vi "EEGteam5.vi"() -> ()   [LabVIEW 2011]
panel:
  in  "stop":bool
  out "After_notch Graph":dynamicdata(graph)
  out "Unfiltered":dynamicdata(graph)
  out "Beta Graph 2":dynamicdata(graph)
  out "Alpha Graph":dynamicdata(graph)
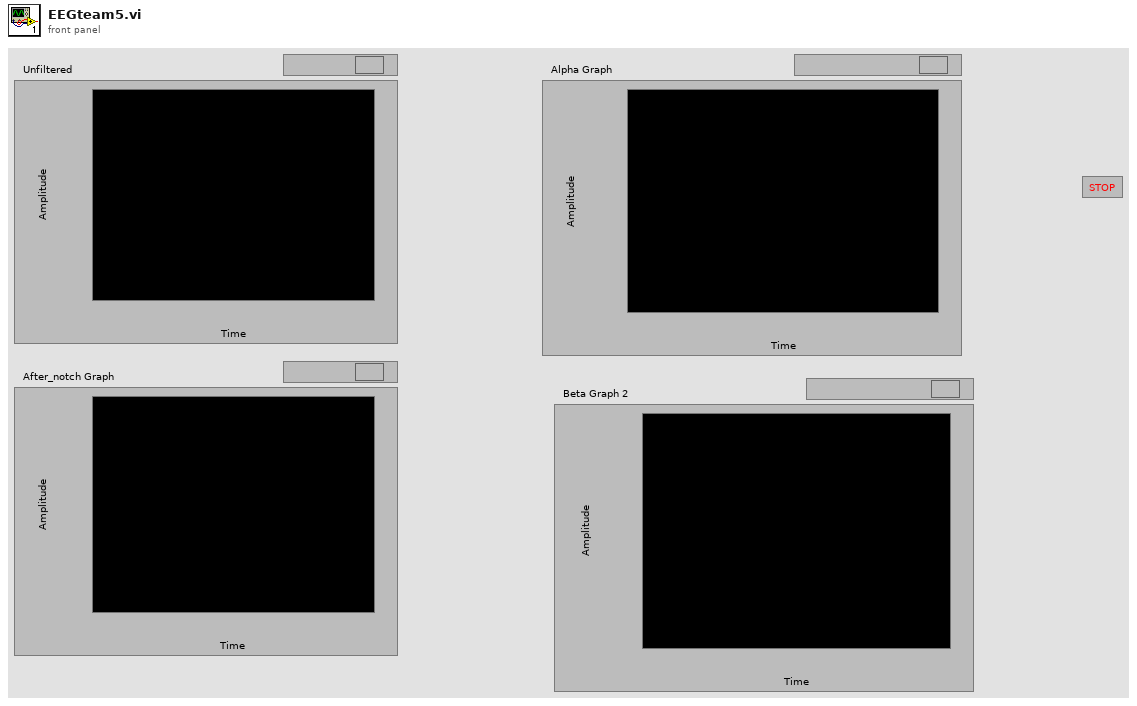
[diagram p1: front panel]
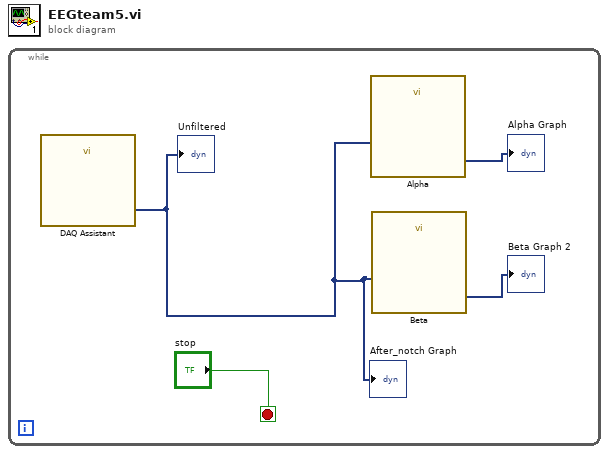
[diagram p0: block diagram]
diagram:
  n1 = while {
    stop <- "stop" stop-if-true
    n2 = call "DAQ Assistant"() -> ("data"=w1:dynamicdata)  [unwired: 17 in, 2 out]
    "Unfiltered" <- w1
    "After_notch Graph" <- w1
    n3 = call "Alpha"("Signal"=w1) -> ("Filtered Signal"=→"Alpha Graph":dynamicdata)  [unwired: 9 in, 1 out]
    n4 = call "Beta"("Signal"=w1) -> ("Filtered Signal"=→"Beta Graph 2":dynamicdata)  [unwired: 9 in, 1 out]
  }
